vi "Update Config Object from File.vi"(8 "error in":errorcluster, 10 "Config File":path, 11 "Config in":refnum<class "Configuration.lvclass">) -> (0 "error out":errorcluster, 3 "Config out":refnum<class "Configuration.lvclass">)   [LabVIEW 2020, in "Logger.lvlib" / "Configuration.lvclass"]
doc: "Given an existing config object, update its configuration cluster from file, preserving all other object data.\n____\nPeloton Config 2.0.0.9\nCopyright (c) 2024, Peloton"
uses:
  Configuration.lvclass
  Configuration.lvclass/Configuration.ctl
  Set Configuration.vi
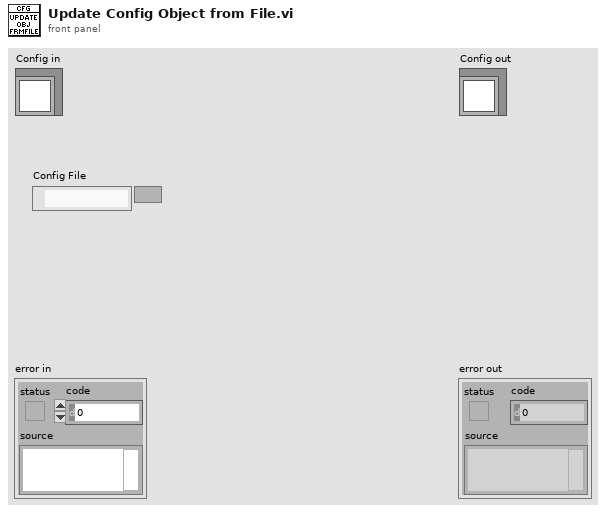
[diagram p1: front panel]
types:
  T1 = typedef "Logger.lvlib/Configuration.lvclass/Configuration--cluster.ctl" = cluster{"File Path":path}
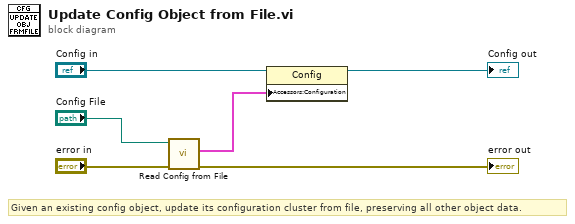
[diagram p0: block diagram]
diagram:
  # "Given an existing config object, update its configuration cluster from file, preserving all other object data."
  n1 = call "Read Config from File.vi"("error in"="error in", "Config File"="Config File") -> ("error out"=→"error out":errorcluster, "Configuration"=w3:T1)  [unwired: 8 in]
  n2 = property class="Config"(reference="Config in", "Accessors:Configuration"=w3) -> (reference out=→"Config out":refnum<class "Configuration.lvclass">)  [unwired: 1 in, 1 out]
